vi "PhotonCamera_SetLEDMode.vi"(9 "LEDMode":T1, 11 "CameraName":string) -> ()   [LabVIEW 2019, in "PhotonVisionLib.lvlib"]
doc: "Sets the LED mode.\n\nInputs:\n - CameraName -- The nickname of the camera (found in the PhotonVision UI).\n - LedMod -- The mode to set to.\n\nOutputs:\n - >none<"
uses:
  PhotonVisionLib.lvlib
  TypeDef/VisionLEDModeType.ctl
  <vilib>/Rock Robotics/Network Tables/NT Write Number.vi
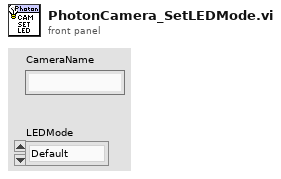
[diagram p1: front panel]
types:
  T1 = typedef "PhotonVisionLib.lvlib/VisionLEDModeType.ctl" = enum16{"Default", "Off", "On", "Blink"}
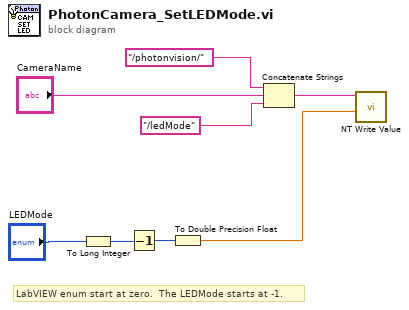
[diagram p0: block diagram]
diagram:
  # "LabVIEW enum start at zero.  The LEDMode starts at -1."
  n1 = To Long Integer(number="LEDMode") -> (32bit integer=w3:i32)
  n2 = Decrement(x=w3) -> (x-1=w2:i32)
  n3 = To Double Precision Float(number=w2) -> (double precision float=w1:dbl)
  n4 = Concatenate Strings("/photonvision/", "CameraName", "/ledMode") -> (w5:string)
  n5 = call-poly <vilib>:"NT Write Value.vi"("Numeric"=w1, "Name"=w5) -> ()  [unwired: 9 in, 1 out]
